vi "LoadController.vi"(8 "error in (no error)":errorcluster, 10 "Actor In":refnum<class "Actor.lvclass">, 11 "DAQ_QPT_Throlab in":refnum<class "DAQ_QPT_Throlab.lvclass">) -> (0 "error out":errorcluster, 3 "DAQ_QPT_Throlab out":refnum<class "DAQ_QPT_Throlab.lvclass">)   [LabVIEW 2020, in "DAQ_QPT_Throlab.lvlib" / "DAQ_QPT_Throlab.lvclass"]
uses:
  DAQ_QPT_Throlab.lvclass
  <vilib>/ActorFramework/Actor/Actor.lvclass
  ViewController/QPDController/QPDController.lvclass
  C:/Program Files/National Instruments/LabVIEW 2020/vi.lib/ActorFramework/Actor/Actor.lvclass
  Hardware Abstraction Layer/Component/DAQ/DAQ/DAQ.lvclass
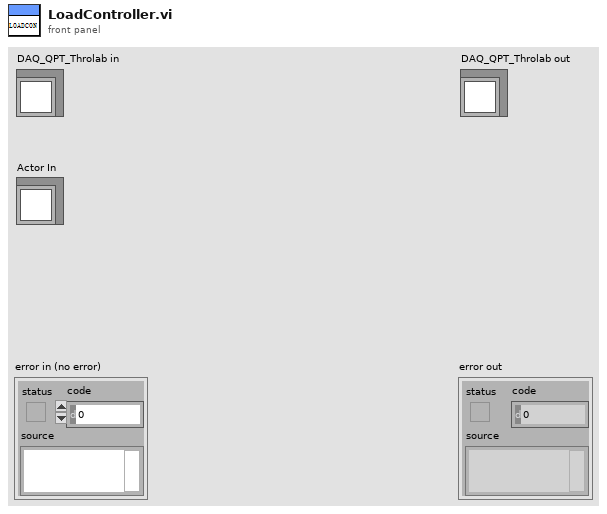
[diagram p1: front panel]
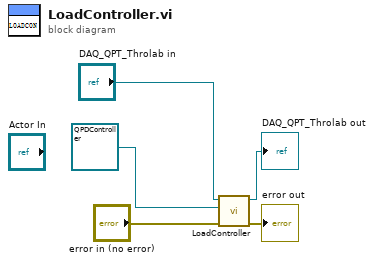
[diagram p0: block diagram]
diagram:
  n1 = call-parent "LoadController.vi"("error in (no error)"="error in (no error)", "Actor In"=refnum<class "QPDController.lvclass"> refnum ("QPDController.lvlib:QPDController.lvclass"), "Device in"="DAQ_QPT_Throlab in") -> ("error out"=→"error out":errorcluster, "Device out"=→"DAQ_QPT_Throlab out":refnum<class "DAQ_QPT_Throlab.lvclass">)  [unwired: 7 in]
